vi "Generate Schema $defs.vi"(8 "error in (no error)":errorcluster, 10 "Object":variant) -> (0 "error out":errorcluster, 2 "Object":variant)   [LabVIEW 2019, in "JSON-Schema.lvlib"]
uses:
  JSON-Schema.lvlib
  <vilib>/Utility/Data Type/NI_Data Type.lvlib
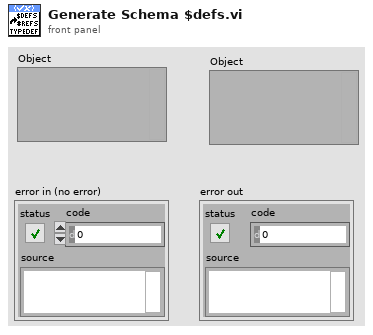
[diagram p1: front panel]
types:
  T1 = typedef "NI_Data Type.lvlib/Data Type.ctl" = enum8{"Invalid Type", "Void", "I8", "I16", "I32", "I64", "U8", "U16", "U32", "U64", "Single Float", "Double Float", "Extended Float", "Single Complex", "Double Complex", "Extended Complex", "Enum U8", "Enum U16", "Enum U32", "Enum U64", "Single Float With Unit", "Double Float With Unit", "Extended Float With Unit", "Single Complex with Unit", "Double Complex with Unit", "Extended Complex with Unit", "Boolean", "String", "Path", "Picture", "Tag", "Array", "Cluster", "Variant", "LV Variant", "Waveform", "Timestamp", "Digital Waveform", "Digital Data", "ExpressData", "Refnum", "External Data", "VI", "Poly VI", "LabVIEW Class Instance", "Fixed Point", "Set Collection", "Map Collection"}
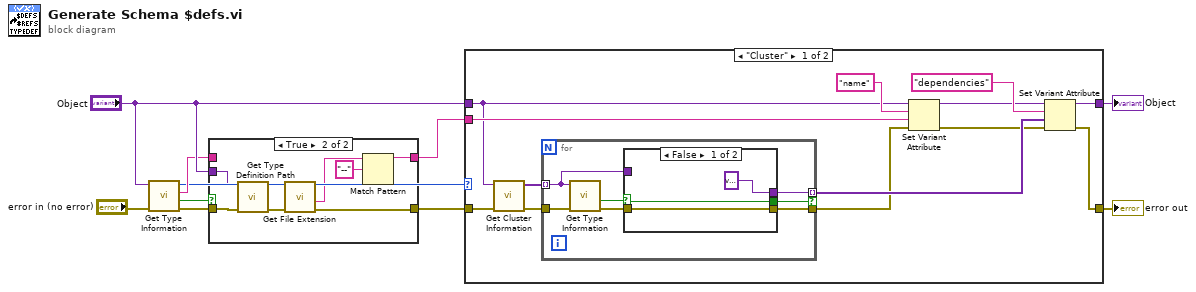
[diagram p0: block diagram]
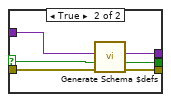
[diagram p2: hidden frame]
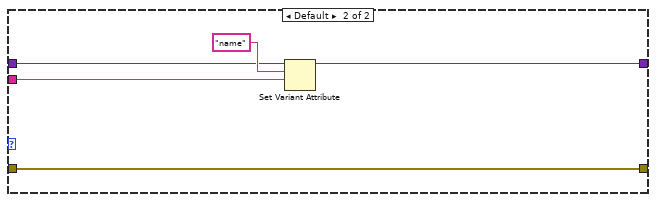
[diagram p3: hidden frame]
diagram:
  n1 = call <vilib>:"Get Type Information.vi"("error in (no error)"="error in (no error)", "variant"="Object") -> ("error out"=w4:errorcluster, "type definition"=w7:bool, "name"=w3:string, "type"=w1:T1)  [unwired: 5 in, 1 out]
  n2 = case shown="True" w7 {
    tunnel: "Object" -> [_ w20]
    tunnel: [w12 w18] -> w5
    tunnel: w4 -> [w11 w15]
    tunnel: w3 -> [w12 _]
    tunnel: [w11 w13] -> w2
    frame False {
    }
    frame True {
      n3 = call <vilib>:"Get Type Definition Path.vi"("error in (no error)"=w15, "variant"=w20) -> ("error out"=w16:errorcluster, "type definition path"=w17:path)  [unwired: 8 in]
      n4 = call <vilib>:"Get File Extension.vi"("error in (no error)"=w16, "file"=w17) -> ("error out"=w13:errorcluster, "filename without extension"=w14:string)  [unwired: 5 in, 3 out]
      n5 = Match Pattern(string=w14, regular expression="--") -> (before substring=w18:string)  [unwired: 1 in, 3 out]
    }
  }
  n6 = case shown="\"Cluster\"" w1 {
    tunnel: "Object" -> [w25 w51]
    tunnel: w2 -> [w31 w53]
    tunnel: [w21 w53] -> w10
    tunnel: w5 -> [w27 w50]
    tunnel: [w24 w49] -> w9
    frame "Cluster" {
      n7 = call <vilib>:"Get Cluster Information.vi"("error in (no error)"=w31, "variant"=w25) -> ("error out"=w32:errorcluster, "cluster elements"=w33:variant[])  [unwired: 8 in]
      n8 = for {
        tunnel: w33 -> [w38] mode=indexing
        tunnel: w32 -> [w40]
        tunnel: [w36] -> w22
        tunnel: [w35] -> w30 mode=indexing if=w34
        n9 = call <vilib>:"Get Type Information.vi"("error in (no error)"=w40, "variant"=w38) -> ("error out"=w37:errorcluster, "type definition"=w39:bool)  [unwired: 5 in, 3 out]
        n10 = case shown="False" w39 {
          selector: w39 -> [w41 w44]
          tunnel: w38 -> [_ w46]
          tunnel: w37 -> [w43 w45]
          tunnel: [w43 w48] -> w36
          tunnel: [variant ("Value") w47] -> w35
          tunnel: [w41 w44] -> w34
          frame False {
          }
          frame True {
            n11 = call "Generate Schema $defs.vi"("error in (no error)"=w45, "Object"=w46) -> ("error out"=w48:errorcluster, "Object"=w47:variant)  [unwired: 8 in]
          }
        }
      }
      n12 = Set Variant Attribute(Variant=w25, name="name", value=w27, error in=w22) -> (Variant out=w26:variant, error out=w23:errorcluster)  [unwired: 1 out]
      n13 = Set Variant Attribute(Variant=w26, name="dependencies", value=w30, error in=w23) -> (Variant out=w24:variant, error out=w21:errorcluster)  [unwired: 1 out]
    }
    frame Default {
      n14 = Set Variant Attribute(Variant=w51, name="name", value=w50) -> (Variant out=w49:variant)  [unwired: 1 in, 2 out]
    }
  }
  "error out" <- w10
  "Object" <- w9
